vi "write.vi"() -> ()   [LabVIEW 2015]
uses:
  Control  rossss.ctl
panel:
  in  "Cluster":cluster{"Topic to write":string, "type":string}={"Topic to write"="rio", "type"="std_msgs/Int32MultiArray"}
  out "Opcode 2":u8
  out "Data 2":string
  out "error out":errorcluster
  in  "rosbridge port":u16=9090
  in  "rosbridge server IP":string="192.168.164.128"
  out "raw JSON frame":string
  in  "stop":bool
  out "concatenated string":string
  in  "format wiadomości":T1={"op"="publish", "topic"="", "msg"={"layout"={"dim"=[], "data_offset"=0.0}, "data"=[]}}
  out "output cluster":T1={"op"="publish", "topic"="", "msg"={"layout"={"dim"=[], "data_offset"=0.0}, "data"=[]}}
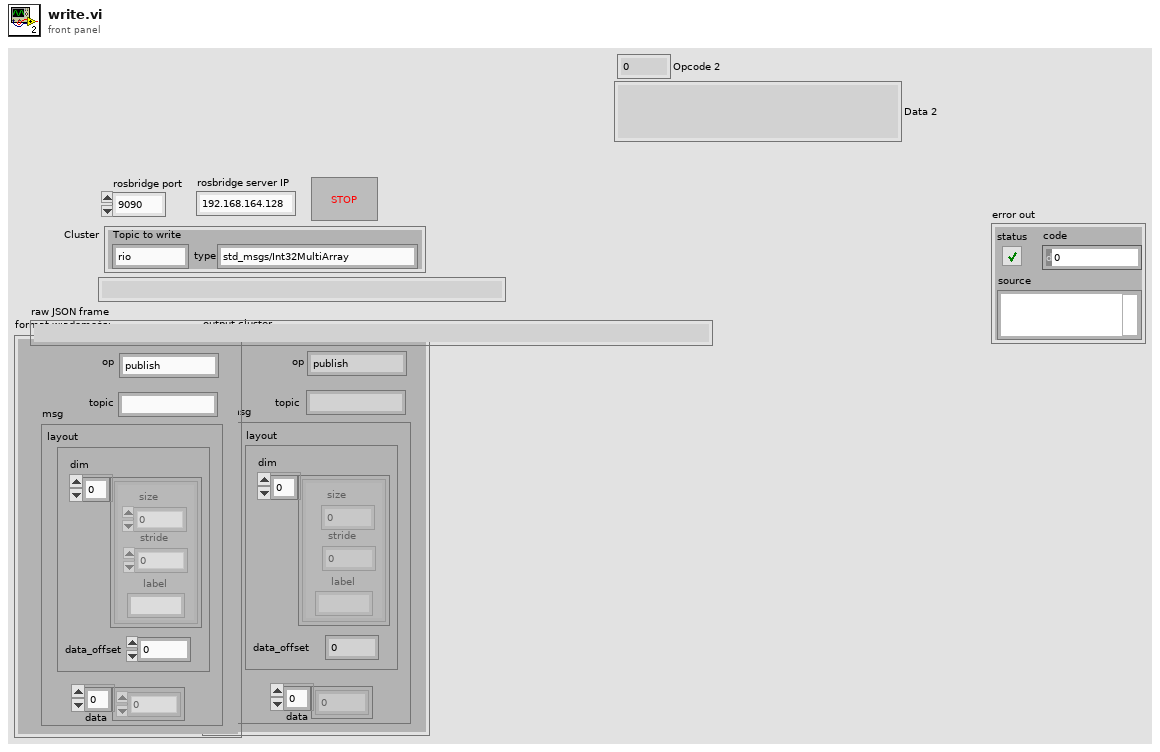
[diagram p1: front panel]
types:
  T1 = typedef "Control  rossss.ctl" = cluster{"op":string, "topic":string, "msg":cluster{"layout":cluster{"dim":cluster{"stride":i16, "size":i16, "label":string}[], "data_offset":dbl}, "data":i32[]}}
  T2 = cluster{"Topic to write":string, "TCP Network Connection out":refnum<k5>, "error out":errorcluster}
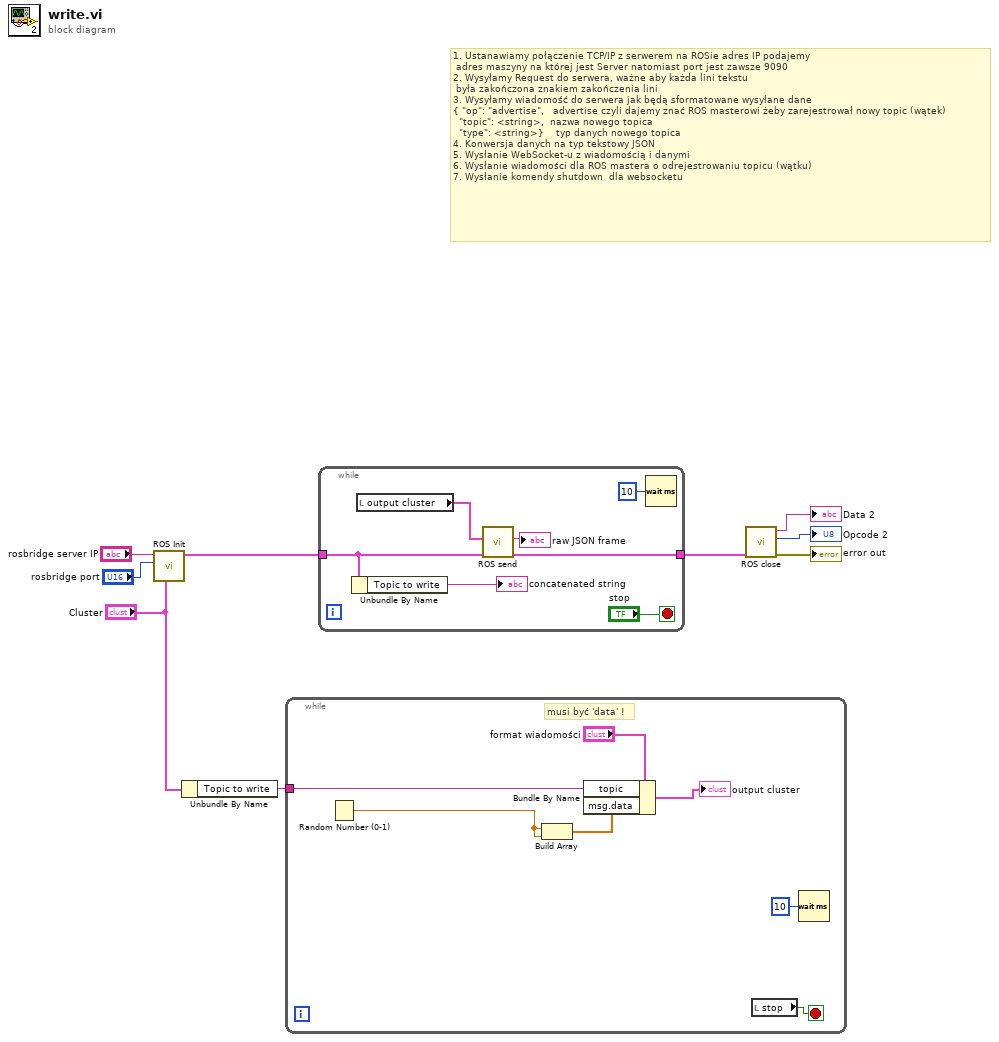
[diagram p0: block diagram]
diagram:
  # "1. Ustanawiamy połączenie TCP/IP z serwerem na ROSie adres IP podajemy\n adres maszyny na której jest Server natomiast port jest zawsze 9090\n2. Wysyłamy Request do serwera, ważne aby każda lini tekstu\n była zakończona znakiem zakończenia lini\n3. Wysyłamy wiadomość do serwera jak będą sformatowane wysyłane dane \n{ \"op\": \"advertise\",   advertise czyli dajemy znać ROS masterowi żeby zarejestrował nowy topic (wątek)\n  \"topic\": <string>,  nazwa nowego topica \n  \"type\": <string>}    typ danych nowego topica\n4. Konwersja danych na typ tekstowy JSON\n5. Wysłanie WebSocket-u z wiadomością i danymi\n6. Wysłanie wiadomości dla ROS mastera o odrejestrowaniu topicu (wątku)\n7. Wysłanie komendy shutdown  dla websocketu"
  n1 = call "ROS Init.vi"("Cluster"="Cluster", "rosbridge port"="rosbridge port", "rosbridge server IP"="rosbridge server IP") -> ("output cluster"=w9:T2)  [unwired: 7 in, 1 out]
  n2 = Unbundle By Name("Cluster") -> ("Topic to write"=w2:string)
  n3 = while {
    tunnel: w2 -> [w14]
    stop <- w15 stop-if-true
    # "musi być 'data' !"
    n4 = Random Number (0-1)() -> (number: 0 to 1=w10:dbl)
    n5 = Build Array(w10, w10) -> (w11:dbl[])
    n6 = Bundle By Name(cluster="format wiadomości", "topic"=w14, "msg.data"=w11) -> (→"output cluster":T1)
    n7 = local read "stop"() -> (w15:bool)
    n8 = Wait (ms)(milliseconds to wait=u32 10) -> ()  [unwired: 1 out]
  }
  n9 = while {
    tunnel: [w23] -> w1
    tunnel: w9 -> [w18]
    stop <- "stop" stop-if-true
    n10 = Unbundle By Name(w18) -> ("Topic to write"=→"concatenated string":string)
    n11 = local read "output cluster"() -> (w19:T1)
    n12 = call "ROS send.vi"("CON IN"=w18, "Data in"=w19) -> ("CON out"=w23:T2, "JSON string"=→"raw JSON frame":string)  [unwired: 8 in]
    n13 = Wait (ms)(milliseconds to wait=u32 10) -> ()  [unwired: 1 out]
  }
  n14 = call "ROS close.vi"("output cluster 2"=w1) -> ("error out"=→"error out":errorcluster, "Opcode 2"=→"Opcode 2":u8, "Data 2"=→"Data 2":string)  [unwired: 8 in]
